vi "ExSubCreateFileMultImage.vi"(0 "Camera Handle":u32, 1 "Pulser Handle":u32, 2 "File and Display Name":string, 3 "error in (no error)":errorcluster, 4 "Number of Images":u32=1 min=1 step=1) -> (5 "Handles Out":T1, 6 "Array":u32[](array[numeric]), 7 "error out":errorcluster)   [LabVIEW 2010]
panel:
  # "ExSubCreateFileMultImage.vi:\nThis is a SubVI that creates a file,  and image objects and returns the handles bundled in a cluster that includes a pulser and camera handle"
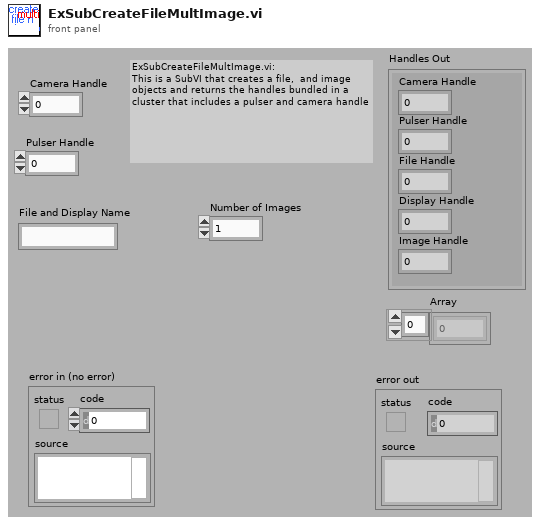
[diagram p1: front panel]
types:
  T1 = cluster{"Camera Handle":u32, "Pulser Handle":u32, "File Handle":u32, "Display Handle":u32, "Image Handle":u32}
  T2 = cluster{"Camera Handle":u32, "Pulser Handle":u32, "File Handle":u32, i32, "Image Handle":u32}
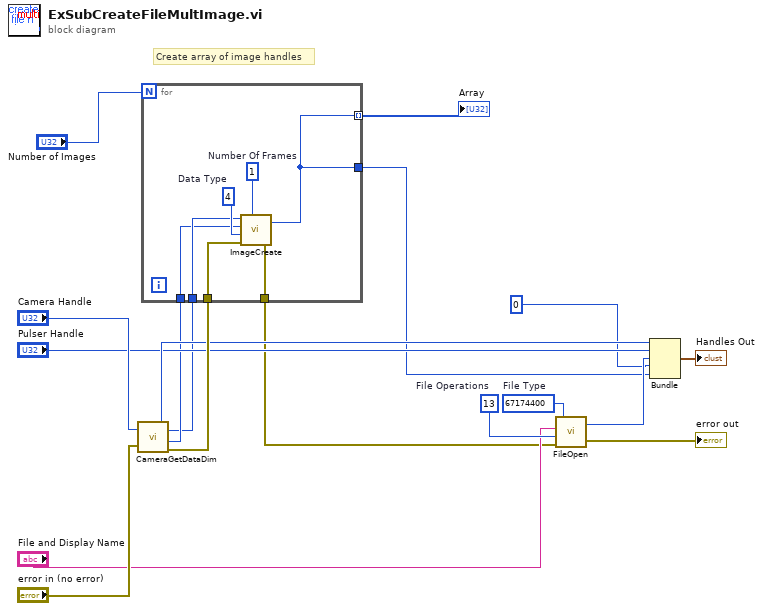
[diagram p0: block diagram]
diagram:
  w9 = 13  # File Operations
  w10 = 67174400  # File Type
  # "Create array of image handles"
  n1 = call <userlib>:"CameraGetDataDim.vi"("Camera Handle"="Camera Handle", "error in"="error in (no error)") -> ("Camera Handle"=w14:u32, "Xdim"=w4:u32, "Ydim"=w5:u32, "error out"=w18:errorcluster)
  n2 = for {
    N: "Number of Images" -> [_]
    tunnel: w18 -> [w25]
    tunnel: [w24] -> w3
    tunnel: [w23] -> w11
    tunnel: w4 -> [w20]
    tunnel: w5 -> [w19]
    tunnel: [w23] -> w6 mode=indexing
    w21 = u32 1  # Number Of Frames
    w22 = u32 4  # Data Type
    n3 = call <userlib>:"ImageCreate.vi"("X dimension"=w20, "Y dimension"=w19, "Data Type"=w22, "error in"=w25, "Number Of Frames"=w21) -> ("Image Handle"=w23:u32, "error out"=w24:errorcluster)
  }
  "Array" <- w6
  n4 = call <userlib>:"FileOpen.vi"("error in"=w3, "File Operations"=w9, "FileName"="File and Display Name", "File Type"=w10) -> ("error out"=→"error out":errorcluster, "File Handle"=w12:u32)
  n5 = Bundle("Camera Handle"=w14, "Pulser Handle"="Pulser Handle", "File Handle"=w12, 0, "Image Handle"=w11) -> (→"Handles Out":T2)  [unwired: 1 in]
